vi "Select Variables.vi"(1 "Variables":T1) -> (0 "Variable Info":T2)   [LabVIEW 2012, in "FEM-03.lvlib"]
uses:
  FEM-03.lvlib
  Controls/Variable Info.ctl
  Controls/Variable List.ctl
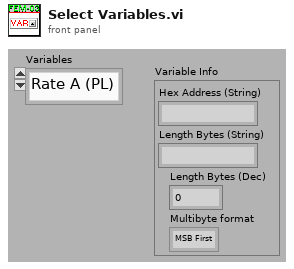
[diagram p1: front panel]
types:
  T1 = typedef "FEM-03.lvlib/Variable List.ctl" = enum16{"Rate A (PL)", "Rate A (GT)", "Job Total A", "Grand Total A", "A-KFR for Rate", "A-KFR decimal point location", "A-KFT for Total", "A-KFT decimal point location ", "A-Rate Engineering Units", "A-Total Engineering units", "A-Flow Direction", "Rate B (PL)", "Rate B (GT)", "Job Total B", "Grand Total B", "B-KFR for Rate", "B-KFR deciminal point location", "B-Rate Engineering units", "B-KFT for Total", "B-KFT decimal point location", "B-Total Engineering units", "Limit 1 Mode", "Limit1", "Margin 1 for rate limit", "Limit 2 Mode", "Limit2", "Margin 2 for rate limit", "Milli-amps Offset", "Milli-amps Out", "Analog Out Mode", "Serial Speed", "Unit Number", "Serial RESET TOTAL", "Update EEPROM", "Relay Override", "FORCE mA Output"}
  T2 = typedef "FEM-03.lvlib/Variable Info.ctl" = cluster{"Hex Address (String)":string, "Length Bytes (String)":string, "Length Bytes (Dec)":i32, "Multibyte format":enum16{"MSB First", "Array last digit 0", "None"}}
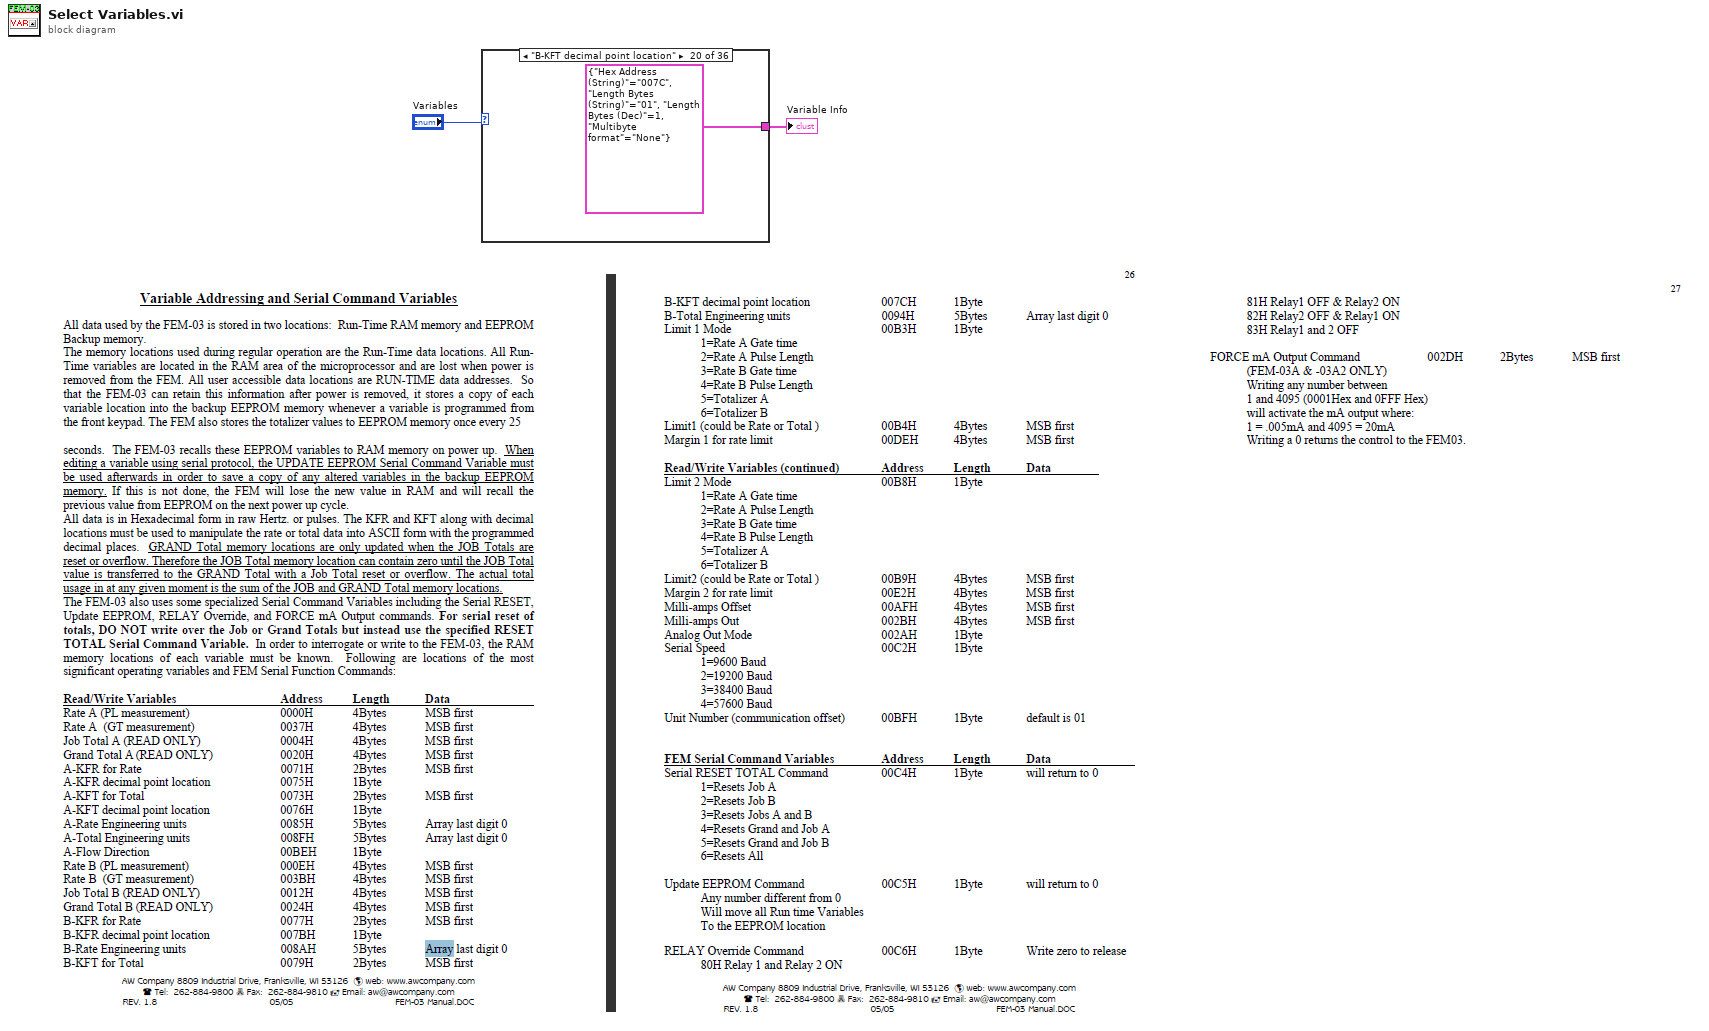
[diagram p0: block diagram]
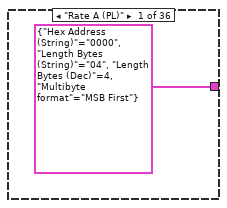
[diagram p2: hidden frame]
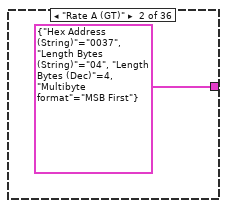
[diagram p3: hidden frame]
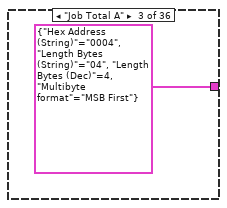
[diagram p4: hidden frame]
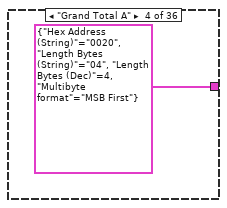
[diagram p5: hidden frame]
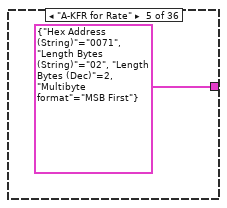
[diagram p6: hidden frame]
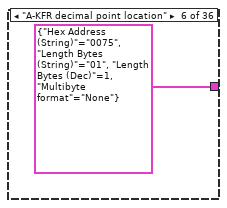
[diagram p7: hidden frame]
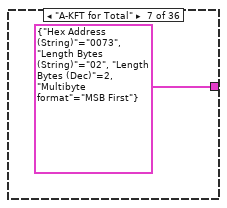
[diagram p8: hidden frame]
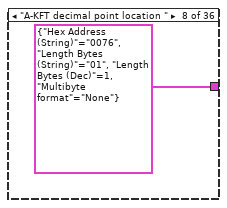
[diagram p9: hidden frame]
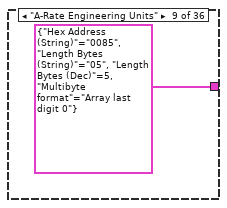
[diagram p10: hidden frame]
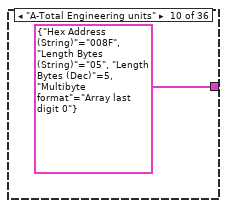
[diagram p11: hidden frame]
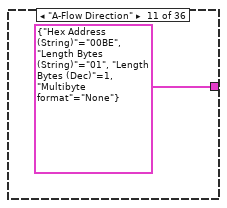
[diagram p12: hidden frame]
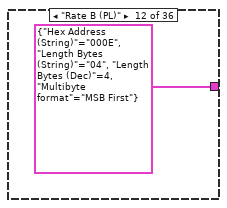
[diagram p13: hidden frame]
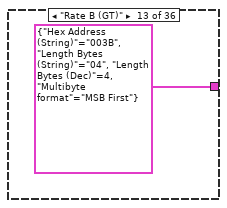
[diagram p14: hidden frame]
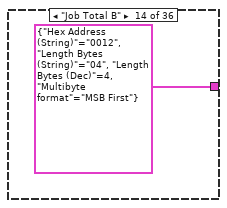
[diagram p15: hidden frame]
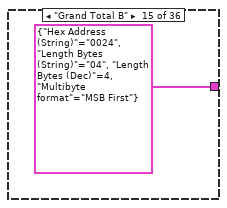
[diagram p16: hidden frame]
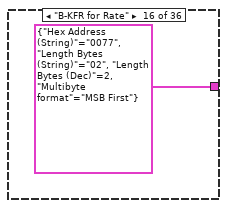
[diagram p17: hidden frame]
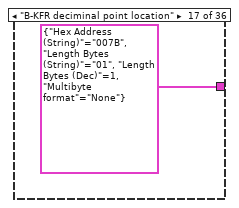
[diagram p18: hidden frame]
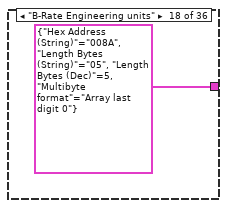
[diagram p19: hidden frame]
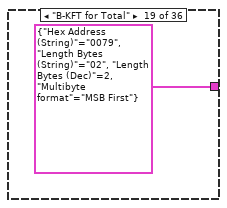
[diagram p20: hidden frame]
diagram:
  n1 = case shown="\"B-KFT decimal point location\"" "Variables" {
    tunnel: [T2 {"Hex Address (String)"="0000", "Length Bytes (String)"="04", "Length Bytes (Dec)"=4, "Multibyte format"=enum."MSB First"} ("Variable Info") T2 {"Hex Address (String)"="0037", "Length Bytes (String)"="04", "Length Bytes (Dec)"=4, "Multibyte format"=enum."MSB First"} ("Variable Info") T2 {"Hex Address (String)"="0004", "Length Bytes (String)"="04", "Length Bytes (Dec)"=4, "Multibyte format"=enum."MSB First"} ("Variable Info") T2 {"Hex Address (String)"="0020", "Length Bytes (String)"="04", "Length Bytes (Dec)"=4, "Multibyte format"=enum."MSB First"} ("Variable Info") T2 {"Hex Address (String)"="0071", "Length Bytes (String)"="02", "Length Bytes (Dec)"=2, "Multibyte format"=enum."MSB First"} ("Variable Info") T2 {"Hex Address (String)"="0075", "Length Bytes (String)"="01", "Length Bytes (Dec)"=1, "Multibyte format"=enum."None"} ("Variable Info") T2 {"Hex Address (String)"="0073", "Length Bytes (String)"="02", "Length Bytes (Dec)"=2, "Multibyte format"=enum."MSB First"} ("Variable Info") T2 {"Hex Address (String)"="0076", "Length Bytes (String)"="01", "Length Bytes (Dec)"=1, "Multibyte format"=enum."None"} ("Variable Info") T2 {"Hex Address (String)"="0085", "Length Bytes (String)"="05", "Length Bytes (Dec)"=5, "Multibyte format"=enum."Array last digit 0"} ("Variable Info") T2 {"Hex Address (String)"="008F", "Length Bytes (String)"="05", "Length Bytes (Dec)"=5, "Multibyte format"=enum."Array last digit 0"} ("Variable Info") T2 {"Hex Address (String)"="00BE", "Length Bytes (String)"="01", "Length Bytes (Dec)"=1, "Multibyte format"=enum."None"} ("Variable Info") T2 {"Hex Address (String)"="000E", "Length Bytes (String)"="04", "Length Bytes (Dec)"=4, "Multibyte format"=enum."MSB First"} ("Variable Info") T2 {"Hex Address (String)"="003B", "Length Bytes (String)"="04", "Length Bytes (Dec)"=4, "Multibyte format"=enum."MSB First"} ("Variable Info") T2 {"Hex Address (String)"="0012", "Length Bytes (String)"="04", "Length Bytes (Dec)"=4, "Multibyte format"=enum."MSB First"} ("Variable Info") T2 {"Hex Address (String)"="0024", "Length Bytes (String)"="04", "Length Bytes (Dec)"=4, "Multibyte format"=enum."MSB First"} ("Variable Info") T2 {"Hex Address (String)"="0077", "Length Bytes (String)"="02", "Length Bytes (Dec)"=2, "Multibyte format"=enum."MSB First"} ("Variable Info") T2 {"Hex Address (String)"="007B", "Length Bytes (String)"="01", "Length Bytes (Dec)"=1, "Multibyte format"=enum."None"} ("Variable Info") T2 {"Hex Address (String)"="008A", "Length Bytes (String)"="05", "Length Bytes (Dec)"=5, "Multibyte format"=enum."Array last digit 0"} ("Variable Info") T2 {"Hex Address (String)"="0079", "Length Bytes (String)"="02", "Length Bytes (Dec)"=2, "Multibyte format"=enum."MSB First"} ("Variable Info") T2 {"Hex Address (String)"="007C", "Length Bytes (String)"="01", "Length Bytes (Dec)"=1, "Multibyte format"=enum."None"} ("Variable Info") T2 {"Hex Address (String)"="0094", "Length Bytes (String)"="05", "Length Bytes (Dec)"=5, "Multibyte format"=enum."Array last digit 0"} ("Variable Info") T2 {"Hex Address (String)"="00B3", "Length Bytes (String)"="01", "Length Bytes (Dec)"=1, "Multibyte format"=enum."None"} ("Variable Info") T2 {"Hex Address (String)"="00B4", "Length Bytes (String)"="04", "Length Bytes (Dec)"=4, "Multibyte format"=enum."MSB First"} ("Variable Info") T2 {"Hex Address (String)"="00DE", "Length Bytes (String)"="04", "Length Bytes (Dec)"=4, "Multibyte format"=enum."MSB First"} ("Variable Info") T2 {"Hex Address (String)"="00B8", "Length Bytes (String)"="01", "Length Bytes (Dec)"=1, "Multibyte format"=enum."None"} ("Variable Info") T2 {"Hex Address (String)"="00B9", "Length Bytes (String)"="04", "Length Bytes (Dec)"=4, "Multibyte format"=enum."MSB First"} ("Variable Info") T2 {"Hex Address (String)"="00E2", "Length Bytes (String)"="04", "Length Bytes (Dec)"=4, "Multibyte format"=enum."MSB First"} ("Variable Info") T2 {"Hex Address (String)"="00AF", "Length Bytes (String)"="04", "Length Bytes (Dec)"=4, "Multibyte format"=enum."MSB First"} ("Variable Info") T2 {"Hex Address (String)"="002B", "Length Bytes (String)"="04", "Length Bytes (Dec)"=4, "Multibyte format"=enum."MSB First"} ("Variable Info") T2 {"Hex Address (String)"="002A", "Length Bytes (String)"="01", "Length Bytes (Dec)"=1, "Multibyte format"=enum."None"} ("Variable Info") T2 {"Hex Address (String)"="00C2", "Length Bytes (String)"="01", "Length Bytes (Dec)"=1, "Multibyte format"=enum."None"} ("Variable Info") T2 {"Hex Address (String)"="00BF", "Length Bytes (String)"="01", "Length Bytes (Dec)"=1, "Multibyte format"=enum."None"} ("Variable Info") T2 {"Hex Address (String)"="00C4", "Length Bytes (String)"="01", "Length Bytes (Dec)"=1, "Multibyte format"=enum."None"} ("Variable Info") T2 {"Hex Address (String)"="00C5", "Length Bytes (String)"="01", "Length Bytes (Dec)"=1, "Multibyte format"=enum."None"} ("Variable Info") T2 {"Hex Address (String)"="00C6", "Length Bytes (String)"="01", "Length Bytes (Dec)"=1, "Multibyte format"=enum."None"} ("Variable Info") T2 {"Hex Address (String)"="002D", "Length Bytes (String)"="02", "Length Bytes (Dec)"=2, "Multibyte format"=enum."MSB First"} ("Variable Info")] -> w2
    frame "Rate A (PL)" {
    }
    frame "Rate A (GT)" {
    }
    frame "Job Total A" {
    }
    frame "Grand Total A" {
    }
    frame "A-KFR for Rate" {
    }
    frame "A-KFR decimal point location" {
    }
    frame "A-KFT for Total" {
    }
    frame "A-KFT decimal point location " {
    }
    frame "A-Rate Engineering Units" {
    }
    frame "A-Total Engineering units" {
    }
    frame "A-Flow Direction" {
    }
    frame "Rate B (PL)" {
    }
    frame "Rate B (GT)" {
    }
    frame "Job Total B" {
    }
    frame "Grand Total B" {
    }
    frame "B-KFR for Rate" {
    }
    frame "B-KFR deciminal point location" {
    }
    frame "B-Rate Engineering units" {
    }
    frame "B-KFT for Total" {
    }
    frame "B-KFT decimal point location" {
    }
    frame "B-Total Engineering units" {
    }
    frame "Limit 1 Mode" {
    }
    frame "Limit1" {
    }
    frame "Margin 1 for rate limit" {
    }
    frame "Limit 2 Mode" {
    }
    frame "Limit2" {
    }
    frame "Margin 2 for rate limit" {
    }
    frame "Milli-amps Offset" {
    }
    frame "Milli-amps Out" {
    }
    frame "Analog Out Mode" {
    }
    frame "Serial Speed" {
    }
    frame "Unit Number" {
    }
    frame "Serial RESET TOTAL" {
    }
    frame "Update EEPROM" {
    }
    frame "Relay Override" {
    }
    frame "FORCE mA Output" {
    }
  }
  "Variable Info" <- w2
